vi "EingabeHilfe.vi"() -> ()   [LabVIEW 2018]
panel:
  in  "Systemdezimalzeichen verwenden (T)":bool
  in  "Inkrement":dbl format="%#_13g"
  in  "Endwert(Exp)":dbl format="%#_13g"
  out "?":string
  in  "Endwert(Fixe Schrittweite)":dbl format="%#_13g"
  in  "Startwert":dbl format="%#_13g"
  in  "Schrittweite":dbl format="%#_13g"
  in  "Feste Schrittweite/Exponentiell":bool=TRUE
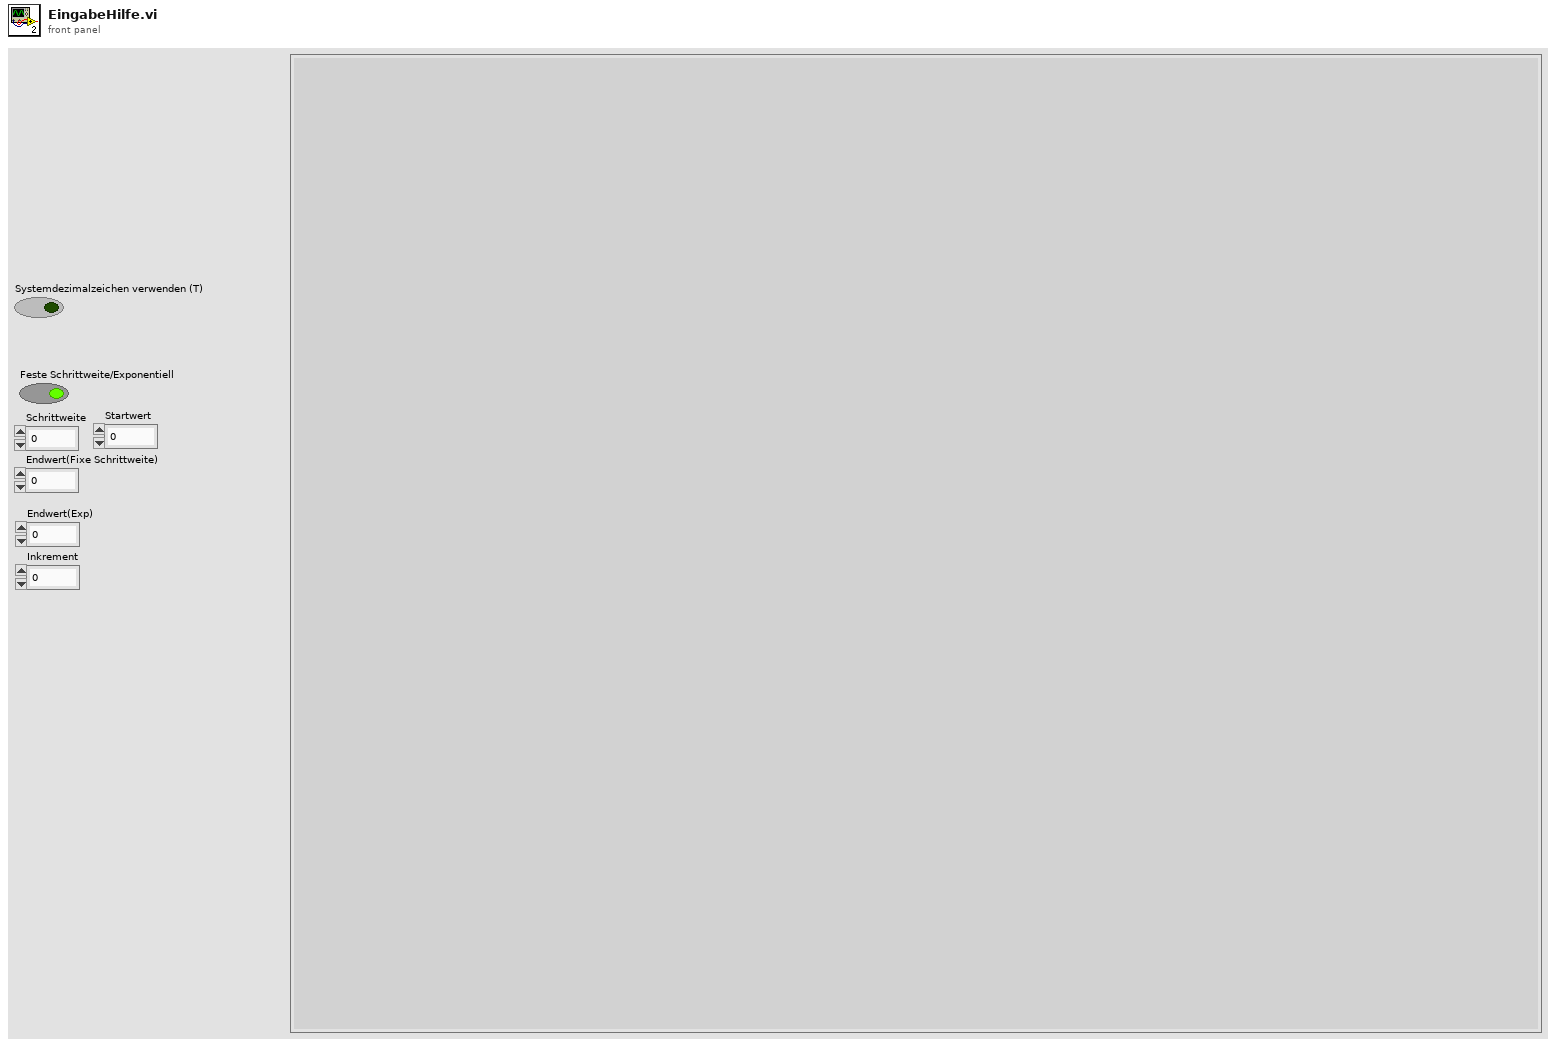
[diagram p1: front panel]
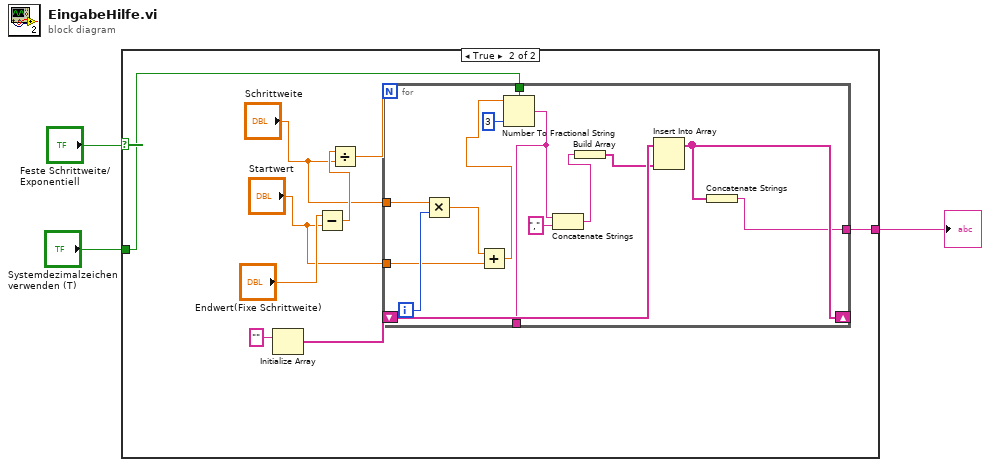
[diagram p0: block diagram]
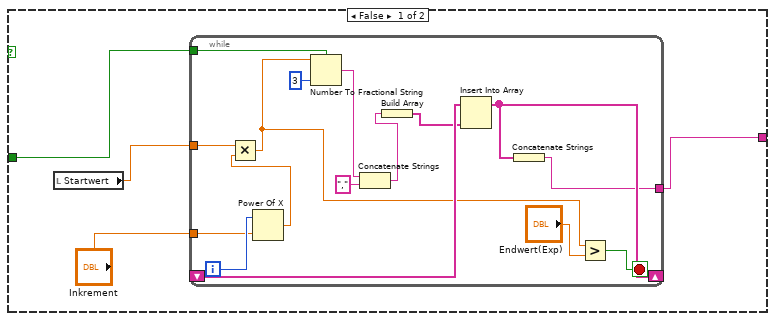
[diagram p2: hidden frame]
diagram:
  n1 = case shown="True" "Feste Schrittweite/Exponentiell" {
    tunnel: [w5 w25] -> w2
    tunnel: "Systemdezimalzeichen verwenden (T)" -> [w4 w24]
    frame False {
      n2 = local read "Startwert"() -> (w7:dbl)
      n3 = while {
        shift-right: [w21] -> _
        shift-left: _ -> [w23]
        tunnel: [w17] -> w5
        tunnel: w7 -> [w14]
        tunnel: "Inkrement" -> [w12]
        tunnel: w4 -> [w9]
        i -> [w13]
        stop <- w16 stop-if-true
        n4 = Power Of X(1:w12, 2:w13) -> (0:w11:dbl)
        n5 = Multiply(x=w14, y=w11) -> (x*y=w10:dbl)
        n6 = Number To Fractional String(use system decimal point (T)=w9, number=w10, precision (6)=i16 3 ("Genauigkeit (6)")) -> (F-format string=w8:string)  [unwired: 1 in]
        n7 = Concatenate Strings(w8, "," ("String")) -> (w19:string)
        n8 = Build Array(w19) -> (w22:string[])
        n9 = Insert Into Array(array=w23, new element=w22) -> (w21:string[])  [unwired: 1 in]
        n10 = Concatenate Strings(w21) -> (w17:string)
        n11 = Greater?(x=w10, y="Endwert(Exp)") -> (0:w16:bool)
      }
    }
    frame True {
      n12 = Initialize Array("" ("Element")) -> (w27:string[])  [unwired: 1 in]
      n13 = Subtract(x="Endwert(Fixe Schrittweite)", y="Startwert") -> (x-y=w31:dbl)
      n14 = Divide(x=w31, y="Schrittweite") -> (x/y=w30:dbl)
      n15 = for {
        N: w30 -> [_]
        tunnel: "Schrittweite" -> [w45]
        tunnel: "Startwert" -> [w43]
        shift-right: [w40] -> _
        shift-left: w27 -> [w42]
        tunnel: [w36] -> _
        tunnel: [w34] -> w25
        tunnel: w24 -> [w33]
        i -> [w46]
        n16 = Multiply(x=w45, y=w46) -> (x*y=w44:dbl)
        n17 = Add(x=w44, y=w43) -> (x+y=w37:dbl)
        n18 = Number To Fractional String(use system decimal point (T)=w33, number=w37, precision (6)=i16 3 ("Genauigkeit (6)")) -> (F-format string=w36:string)  [unwired: 1 in]
        n19 = Concatenate Strings(w36, "," ("String")) -> (w38:string)
        n20 = Build Array(w38) -> (w41:string[])
        n21 = Insert Into Array(array=w42, new element=w41) -> (w40:string[])  [unwired: 1 in]
        n22 = Concatenate Strings(w40) -> (w34:string)
      }
    }
  }
  "?" <- w2
